vi "set Defer FP Updates.vi"(8 "error in (no error)":errorcluster, 10 "Defer FP Updates":bool, 11 "Actor in":refnum<class "Actor.lvclass">) -> (0 "error out":errorcluster)   [LabVIEW 2015, in "Actor.lvclass"]
uses:
  Actor.lvclass
  Actor.lvclass/Actor.ctl
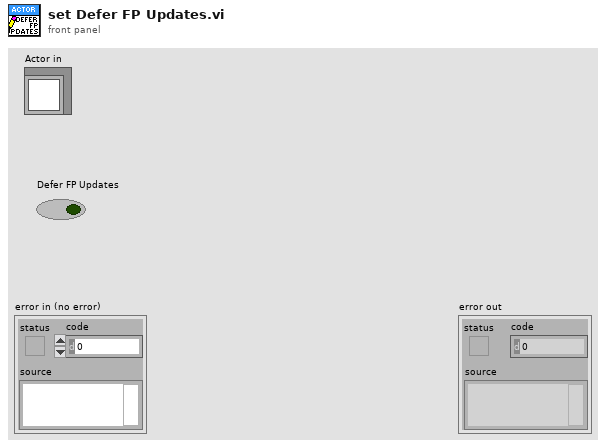
[diagram p1: front panel]
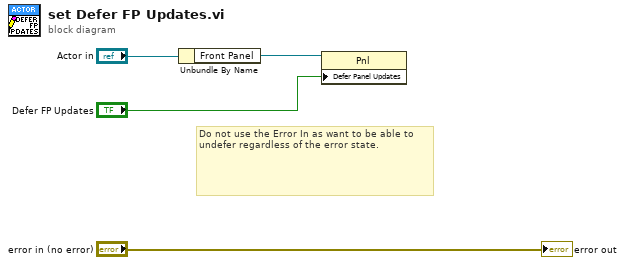
[diagram p0: block diagram]
diagram:
  # "Do not use the Error In as want to be able to undefer regardless of the error state."
  n1 = Unbundle By Name("Actor in") -> ("Front Panel"=w3:refnum<vi>)
  n2 = property class="Pnl"(reference=w3, "Defer Panel Updates"="Defer FP Updates") -> ()  [unwired: 1 in, 2 out]
  "error out" <- "error in (no error)"
